vi "Stitching-Save stitched image.vi"(8 "error in (no error)":errorcluster, 9 "Z-plane":i32, 10 "Base directory containing all dataset folders":path, 11 "Stitched image ref in":T1) -> (0 "error out":errorcluster, 1 "Collage folder":path, 3 "Stitched image ref":T1)   [LabVIEW 2013]
uses:
  <vilib>/vision/Image Controls.llb/IMAQ Image.ctl
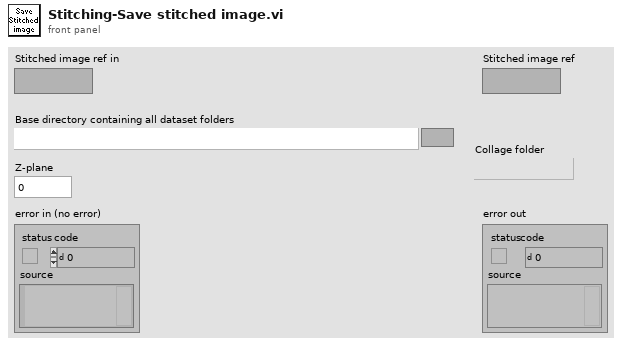
[diagram p1: front panel]
types:
  T1 = typedef "IMAQ Image.ctl" = refnum<image>
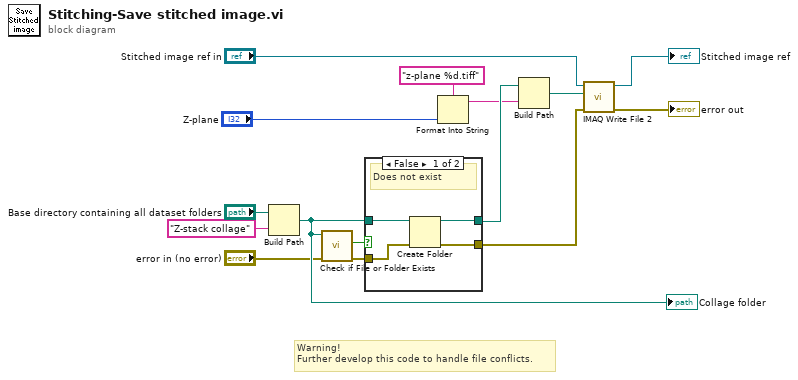
[diagram p0: block diagram]
diagram:
  # "Warning!\nFurther develop this code to handle file conflicts."
  n1 = Build Path(base path="Base directory containing all dataset folders", name or relative path="Z-stack collage") -> (appended path=w10:path)
  "Collage folder" <- w10
  n2 = call <vilib>:"Check if File or Folder Exists.vi"("error in (no error)"="error in (no error)", "path"=w10) -> ("error out"=w9:errorcluster, "file or folder exists?"=w11:bool)  [unwired: 7 in, 1 out]
  n3 = case shown="False" w11 {
    tunnel: w10 -> [w19 w20]
    tunnel: w9 -> [w18 w21]
    tunnel: [w17 w20] -> w7
    tunnel: [w16 w21] -> w2
    frame False {
      # "Does not exist"
      n4 = Create Folder(path (use dialog)=w19, error in=w18) -> (created path=w17:path, error out=w16:errorcluster)  [unwired: 1 in, 1 out]
    }
    frame True {
      # "Exists"
    }
  }
  n5 = Format Into String(format string="z-plane %d.tiff", "Z-plane") -> (resulting string=w4:string)  [unwired: 2 in, 1 out]
  n6 = Build Path(base path=w7, name or relative path=w4) -> (appended path=w6:path)
  n7 = call-poly "IMAQ Write File 2"("error in (no error)"=w2, "File Path"=w6, "Image"="Stitched image ref in") -> ("error out"=→"error out":errorcluster, "Image Out (duplicate)"=→"Stitched image ref":T1)  [unwired: 7 in]
